vi "Engine Display v1.1.vi"(6 "Boolean in":refnum<vi>, 8 "Data In":refnum<notifier>) -> ()   [LabVIEW 2020]
panel:
  out "x/y":dbl
  out "Notif":string
  out "Meter":dbl(knob) scale=50.0..3000.0
  out "PT-CC-410":dbl
  out "TC-CC-412":dbl
  out "TC-CC-411":dbl
  out "TC-CC-410":dbl
  out "Horizontal Graduated Bar":dbl(slide) caption="Meter" scale=0.0..1000.0
  out "Countdown":ext format="%<%M:%S>t"
  out "Thermometer 3":dbl(slide) scale=-300.0..310.0
  out "Thermometer 2":dbl(slide) scale=-300.0..310.0
  out "Thermometer":dbl(slide) scale=-300.0..310.0
  out "LC-CC-410":dbl
  out "Engine Thrust":dbl[](graph)
  # "T"
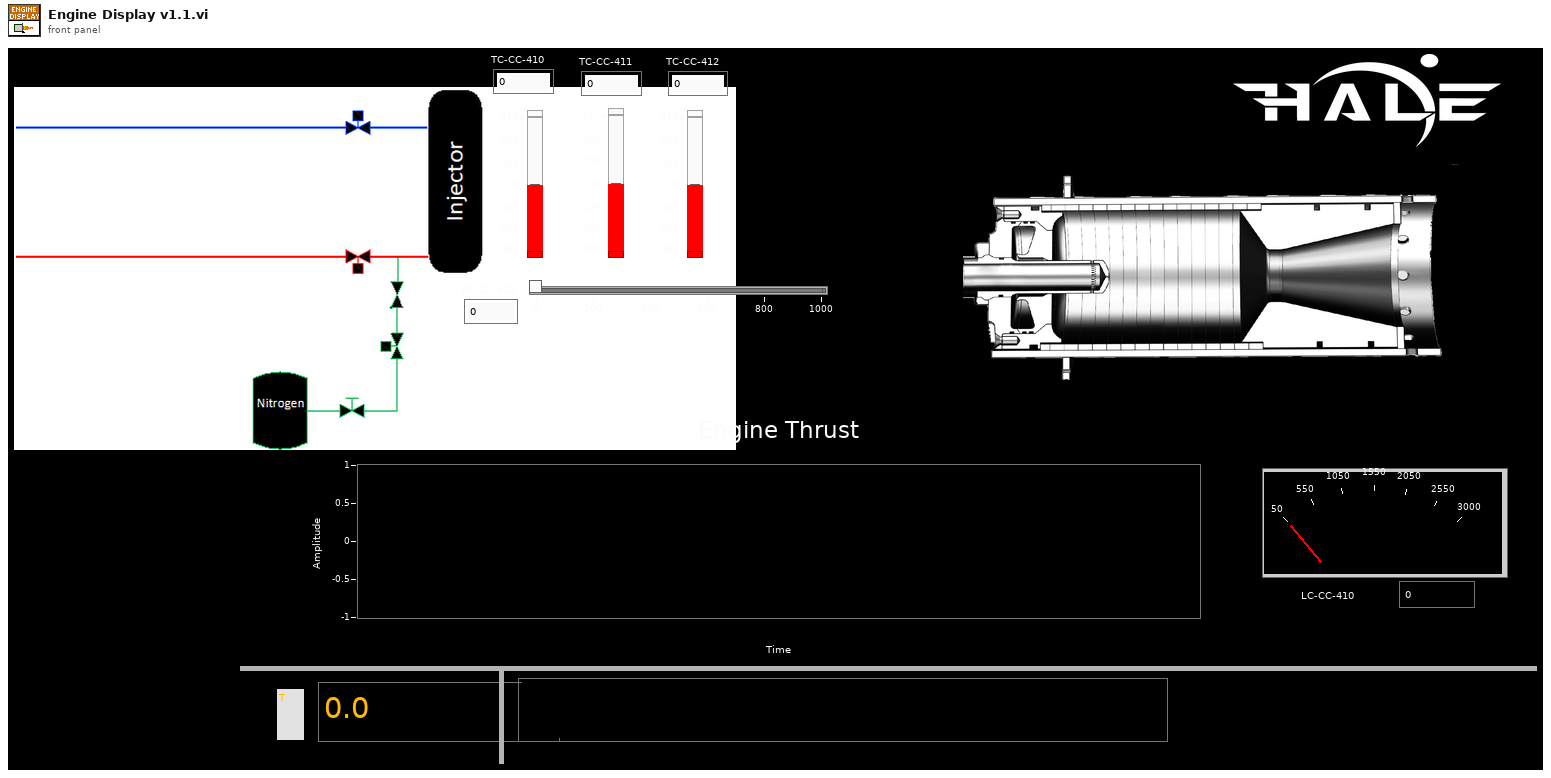
[diagram p1: front panel]
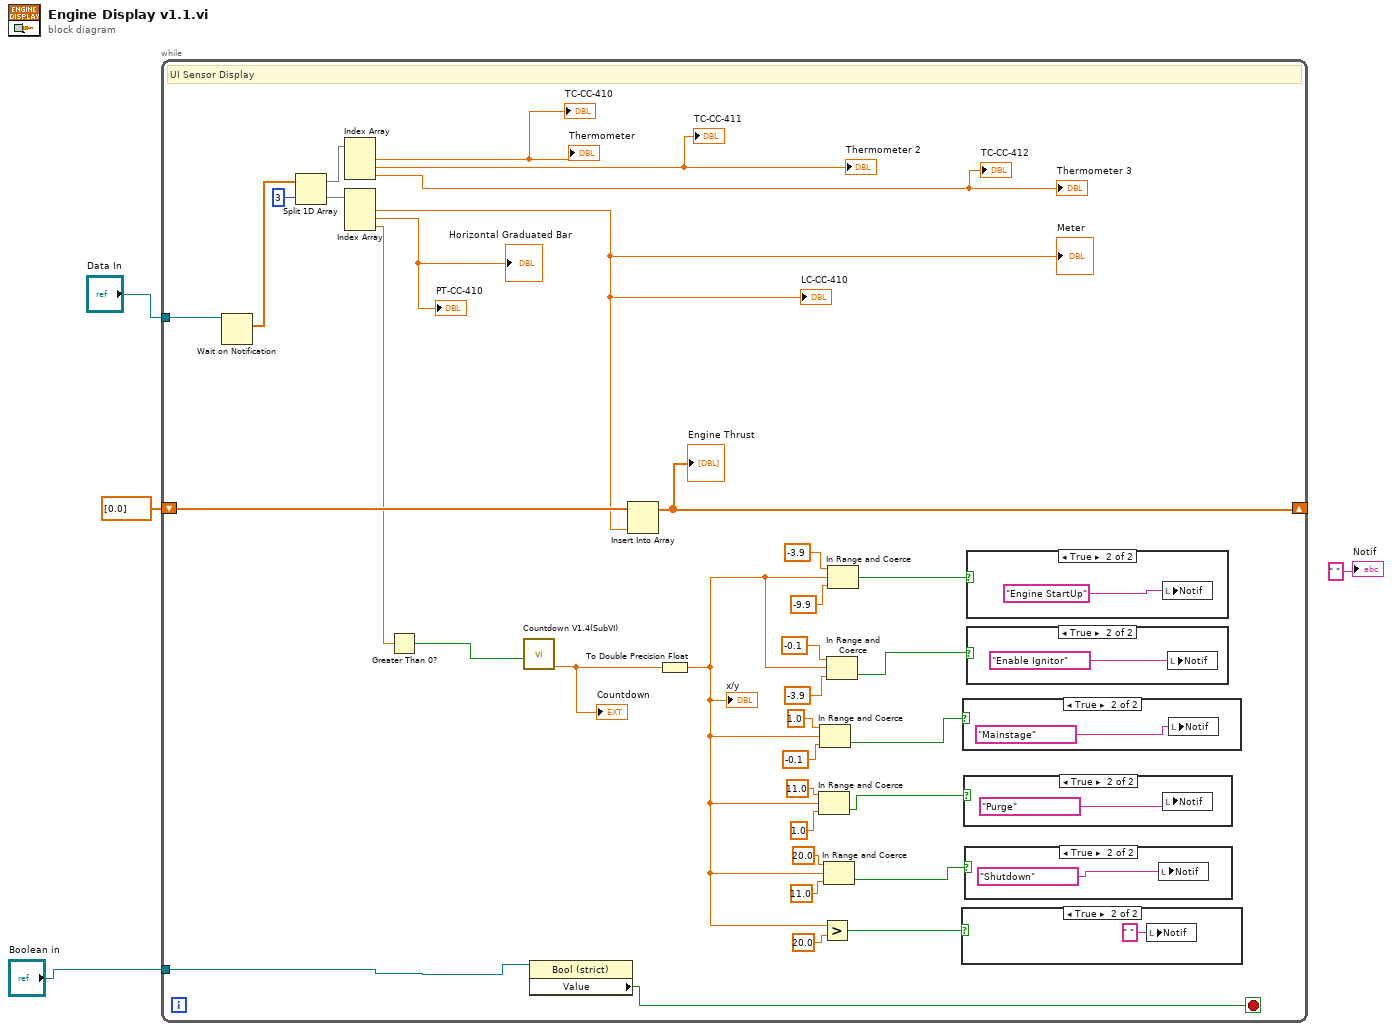
[diagram p0: block diagram]
diagram:
  n1 = while {
    shift-right: [w34] -> _
    shift-left: dbl[] [0.0] -> [w39]
    tunnel: "Data In" -> [w38]
    tunnel: "Boolean in" -> [w6]
    stop <- w5 stop-if-true
    # "UI Sensor Display"
    n2 = Wait on Notification(notifier=w38) -> (notification=w27:dbl[])  [unwired: 3 in, 3 out]
    n3 = Split 1D Array(array=w27, index=3) -> (first subarray=w33:dbl[], second subarray=w36:dbl[])
    n4 = Index Array(array=w33) -> (element #1=→"Thermometer" →"TC-CC-410":dbl, element #2=→"Thermometer 2" →"TC-CC-411":dbl, element #3=→"Thermometer 3" →"TC-CC-412":dbl)  [unwired: 3 in]
    n5 = Index Array(array=w36) -> (element #1=w28:dbl, element #2=→"PT-CC-410" →"Horizontal Graduated Bar":dbl, element #3=w35:dbl)  [unwired: 3 in]
    "LC-CC-410" <- w28
    "Meter" <- w28
    n6 = Greater Than 0?(x=w35) -> (x > 0?=w8:bool)
    n7 = call "Countdown V1.4(SubVI).vi"("start input"=w8) -> ("timer out"=w7:dbl)  [unwired: 10 in]
    "Countdown" <- w7
    n8 = property class="Bool (strict)"(reference=w6) -> ("Value"=w5:bool)  [unwired: 1 in, 2 out]
    n9 = Insert Into Array(array=w39, new element=w28) -> (w34:dbl[])  [unwired: 1 in]
    "Engine Thrust" <- w34
    n10 = To Double Precision Float(number=w7) -> (double precision float=w9:dbl)
    "x/y" <- w9
    n11 = In Range and Coerce(upper limit=11.0, x=w9, lower limit=1.0) -> (In Range?=w12:bool)  [unwired: 1 out]
    n12 = In Range and Coerce(upper limit=1.0, x=w9, lower limit=-0.1) -> (In Range?=w16:bool)  [unwired: 1 out]
    n13 = Greater?(x=w9, y=20.0) -> (0:w11:bool)
    n14 = In Range and Coerce(upper limit=20.0, x=w9, lower limit=11.0) -> (In Range?=w13:bool)  [unwired: 1 out]
    n15 = In Range and Coerce(upper limit=-0.1, x=w9, lower limit=-3.9) -> (In Range?=w21:bool)  [unwired: 1 out]
    n16 = In Range and Coerce(upper limit=-3.9, x=w9, lower limit=-9.9) -> (In Range?=w24:bool)  [unwired: 1 out]
    n17 = case shown="True" w11 {
      frame False {
      }
      frame True {
        n18 = local write "Notif"(" " ("Notif")) -> ()
      }
    }
    n19 = case shown="True" w16 {
      frame False {
      }
      frame True {
        n20 = local write "Notif"("Mainstage") -> ()
      }
    }
    n21 = case shown="True" w12 {
      frame False {
      }
      frame True {
        n22 = local write "Notif"("Purge") -> ()
      }
    }
    n23 = case shown="True" w13 {
      frame False {
      }
      frame True {
        n24 = local write "Notif"("Shutdown") -> ()
      }
    }
    n25 = case shown="True" w24 {
      frame False {
      }
      frame True {
        n26 = local write "Notif"("Engine StartUp") -> ()
      }
    }
    n27 = case shown="True" w21 {
      frame False {
      }
      frame True {
        n28 = local write "Notif"("Enable Ignitor") -> ()
      }
    }
  }
  "Notif" <- " " ("Notif")
